vi "Launch GUI.vi"(8 "error in (no error)":errorcluster, 9 "Sub Panel":refnum<vi>, 10 "GUI Class Path":path, 11 "CS++BaseActor":refnum<class "CS++BaseActor.lvclass">) -> (0 "error out":errorcluster, 3 "CS++BaseActor":refnum<class "CS++BaseActor.lvclass">)   [LabVIEW 2013, in "CS++BaseActor.lvlib" / "CS++BaseActor.lvclass"]
doc: "Launch GUI for this actor."
uses:
  CS++BaseActor.lvclass
  CS++GUIActor/CS++GUIActor.lvclass
  CS++BaseActor.lvclass/CS++BaseActor.ctl
  <vilib>/ActorFramework/Actor/Actor.lvclass/Actor.ctl
  <vilib>/ActorFramework/Message Enqueuer/Message Enqueuer.lvclass/Message Enqueuer.ctl
  CS++GUIActor/CS++GUIActor.lvclass/CS++GUIActor.ctl
  <vilib>/ActorFramework/Message Enqueuer/Init from Existing Queue.vi
  <vilib>/ActorFramework/Message Enqueuer/Message Enqueuer.lvclass
  <vilib>/ActorFramework/Actor/Actor.lvclass
  CS++BaseActor Messages/Open Actor Core FP Msg/Open Actor Core FP Msg.lvclass
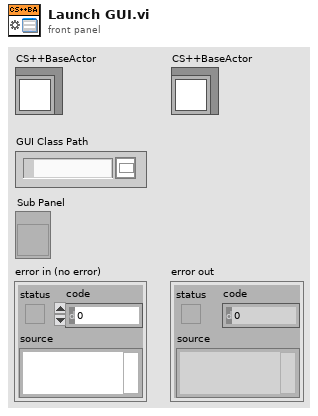
[diagram p1: front panel]
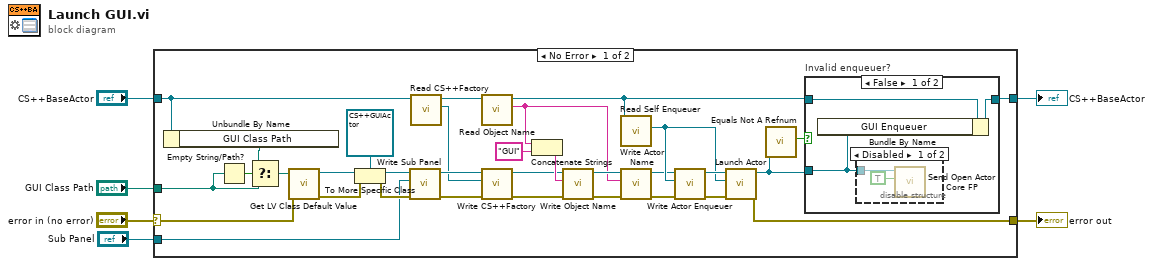
[diagram p0: block diagram]
diagram:
  n1 = case shown="No Error" "error in (no error)" {
    selector: "error in (no error)" -> [w35 w47]
    tunnel: [w30 w47] -> w5
    tunnel: [w31 w46] -> w3
    tunnel: "CS++BaseActor" -> [w13 w46]
    tunnel: "GUI Class Path" -> [w37 _]
    tunnel: "Sub Panel" -> [w25 _]
    frame No Error {
      n2 = Unbundle By Name(w13) -> ("GUI Class Path"=w38:path)
      n3 = Empty String/Path?(string/path=w37) -> (empty?=w39:bool)
      n4 = Select(t=w38, s=w39, f=w37) -> (s? t:f=w36:path)
      n5 = call <vilib>:"Get LV Class Default Value.vi"("error in (no error)"=w35, "class path"=w36) -> ("error out"=w33:errorcluster, "object"=w34:refnum<class>)  [unwired: 8 in]
      n6 = To More Specific Class(target class=refnum<class "CS++GUIActor.lvclass"> refnum ("CS++DeviceGUIActor.lvlib:CS++DeviceGUIActor.lvclass"), reference=w34, error in=w33) -> (specific class reference=w27:refnum<class "CS++GUIActor.lvclass">, error out=w26:errorcluster)
      n7 = call "Write Sub Panel.vi"("error in (no error)"=w26, "Sub Panel"=w25, "CS++DeviceGUIActor in"=w27) -> ("error out"=w9:errorcluster, "CS++DeviceGUIActor out"=w11:refnum<class "CS++GUIActor.lvclass">)  [unwired: 7 in]
      n8 = call "Read CS++Factory.vi"("CS++BaseActor in"=w13) -> ("CS++Factory"=w7:refnum<class "CS++Factory.lvclass">, "CS++BaseActor out"=w12:refnum<class "CS++BaseActor.lvclass">)  [unwired: 8 in, 1 out]
      n9 = call "Read Object Name.vi"("CS++BaseActor in"=w12) -> ("Object Name"=w16:string, "CS++BaseActor out"=w19:refnum<class "CS++BaseActor.lvclass">)  [unwired: 8 in, 1 out]
      n10 = call "Write CS++Factory.vi"("error in (no error)"=w9, "CS++Factory"=w7, "CS++BaseActor in"=w11) -> ("error out"=w8:errorcluster, "CS++BaseActor out"=w10:refnum<class "CS++GUIActor.lvclass">)  [unwired: 7 in]
      n11 = Concatenate Strings(w16, "GUI" ("string")) -> (w14:string)
      n12 = call "Write Object Name.vi"("error in (no error)"=w8, "Object Name"=w14, "CS++BaseActor in"=w10) -> ("error out"=w17:errorcluster, "CS++BaseActor out"=w18:refnum<class "CS++GUIActor.lvclass">)  [unwired: 7 in]
      n13 = call <vilib>:"Read Self Enqueuer.vi"("Actor"=w19) -> ("Self Enqueuer"=w22:refnum<class "Message Enqueuer.lvclass">)  [unwired: 10 in]
      n14 = call "Write Actor Name.vi"("error in (no error)"=w17, "Actor Name"=w16, "CS++DeviceGUIActor in"=w18) -> ("error out"=w20:errorcluster, "CS++DeviceGUIActor out"=w21:refnum<class "CS++GUIActor.lvclass">)  [unwired: 7 in]
      n15 = call "Write Actor Enqueuer.vi"("error in (no error)"=w20, "Actor Enqueuer"=w22, "CS++DeviceGUIActor in"=w21) -> ("error out"=w23:errorcluster, "CS++DeviceGUIActor out"=w24:refnum<class "CS++GUIActor.lvclass">)  [unwired: 7 in]
      n16 = call <vilib>:"Launch Actor.vi"("error in (no error)"=w23, "Actor-to-Caller Enqueuer"=w22, "Actor"=w24) -> ("error out"=w30:errorcluster, "Caller-To-Actor Enqueuer"=w29:refnum<class "Message Enqueuer.lvclass">)  [unwired: 7 in]
      n17 = call <vilib>:"Equals Not A Refnum.vi"("Message Enqueuer"=w29) -> ("Not a refnum?"=w28:bool)  [unwired: 10 in]
      n18 = case "Invalid enqueuer?" shown="False" w28 {
        tunnel: w19 -> [w42 w45]
        tunnel: [w41 w45] -> w31
        tunnel: w29 -> [w40 _]
        frame False {
          n19 = Bundle By Name(cluster=w42, "GUI Enqueuer"=w40) -> (w41:refnum<class "CS++BaseActor.lvclass">)
          n20 = disable-structure shown="Disabled" {
            disable-tunnel: w40 -> [w44 _]
            frame Disabled {
              n21 = call "Send Open Actor Core FP.vi"("Open FP (F)"=TRUE, "Message Enqueuer"=w44) -> ()  [unwired: 8 in, 2 out]
            }
            frame Enabled {
            }
          }
        }
        frame True {
        }
      }
    }
    frame Error {
    }
  }
  "error out" <- w5
  "CS++BaseActor" <- w3
